vi "lv_mysql_conn_ok_packet.vi"(9 "OK Packet Data In":T1 {"Server Status" format="%.0x"}, 11 "TCPIP Data":u8[](array[numeric])) -> (1 "OK Packet Data":T1 {"Server Status" format="%.0x"})   [LabVIEW 2020]
uses:
  typedefs/ok_packet_metadata.ctl
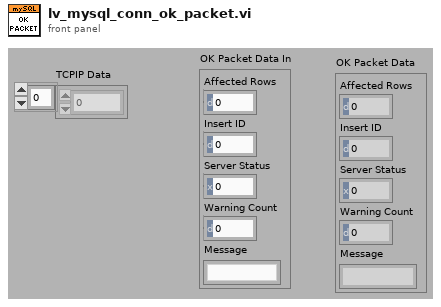
[diagram p1: front panel]
types:
  T1 = typedef "ok_packet_metadata.ctl" = cluster{"Affected Rows":u64, "Insert ID":u64, "Server Status":u16, "Warning Count":u16, "Message":string}
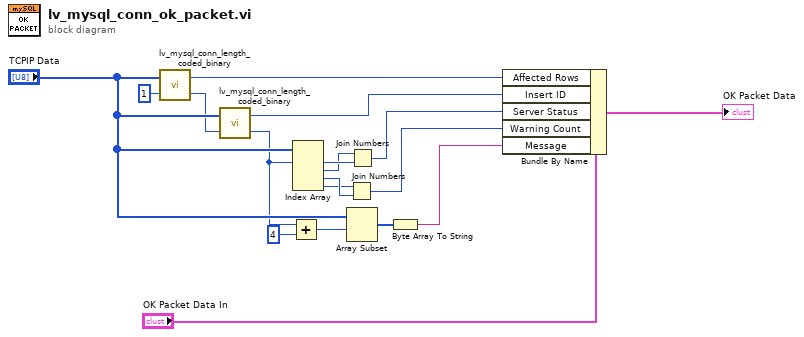
[diagram p0: block diagram]
diagram:
  n1 = call "lv_mysql_conn_length_coded_binary.vi"("Start Index"=1, "Data"="TCPIP Data") -> ("Next Index"=w14:i32, "Output"=w16:u64)
  n2 = call "lv_mysql_conn_length_coded_binary.vi"("Start Index"=w14, "Data"="TCPIP Data") -> ("Next Index"=w5:i32, "Output"=w13:u64)
  n3 = Add(x=w5, y=4) -> (x+y=w6:i32)
  n4 = Index Array(array="TCPIP Data", index #1=w5) -> (element #1=w12:u8, element #2=w11:u8, element #3=w9:u8, element #4=w8:u8)  [unwired: 3 in]
  n5 = Join Numbers(hi=w8, lo=w9) -> ((hi.lo)=w7:u16)
  n6 = Array Subset(array="TCPIP Data", index=w6) -> (w3:u8[])  [unwired: 1 in]
  n7 = Join Numbers(hi=w11, lo=w12) -> ((hi.lo)=w10:u16)
  n8 = Byte Array To String(unsigned byte array=w3) -> (string=w2:string)
  n9 = Bundle By Name(cluster="OK Packet Data In", "Affected Rows"=w16, "Insert ID"=w13, "Server Status"=w10, "Warning Count"=w7, "Message"=w2) -> (→"OK Packet Data":T1)
